vi "DHT11 Example.vi"() -> ()   [LabVIEW 2009, in "DHTXX.lvlib"]
uses:
  DHTXX.lvlib
  <vilib>/LabVIEW Interface for Arduino/LabVIEW Interface for Arduino.lvlib
panel:
  out "OK":bool
  in  "stop":bool
  out "Relative Humidity (%)":dbl(slide)
  out "Temperature (°C)":dbl(slide)
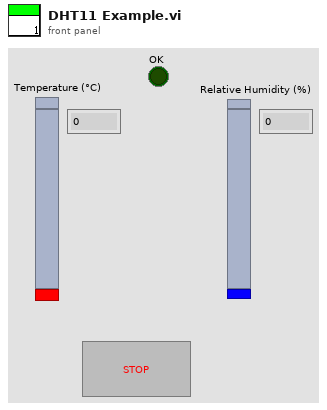
[diagram p1: front panel]
types:
  T1 = typedef "LabVIEW Interface for Arduino.lvlib/Arduino Resource.ctl" = cluster{"VISA resource":refnum<visa-resource-name>, "Board Type":T2, "Connection Type":enum8{"USB / Serial"}, "Bytes Per Packet (15)":u8}
  T2 = typedef "LabVIEW Interface for Arduino.lvlib/Board Type.ctl" = enum16{"Uno", "Dimuelanove w/Atmega 328", "Mega 2560"}
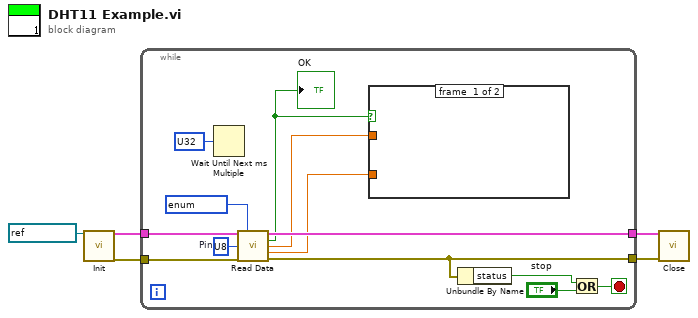
[diagram p0: block diagram]
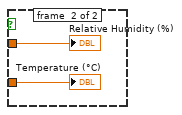
[diagram p2: hidden frame]
diagram:
  n1 = call <vilib>:"Init.vi"("VISA resource"=refnum<visa-resource-name> ?) -> ("Arduino Resource"=w5:T1, "error out"=w4:errorcluster)  [unwired: 17 in]
  n2 = while {
    tunnel: w5 -> [w18]
    tunnel: w4 -> [w17]
    tunnel: [w16] -> w3
    tunnel: [w8] -> w2
    stop <- w12 stop-if-true
    w9 = u8 ?  # Pin
    n3 = Wait Until Next ms Multiple(millisecond multiple=u32 ?) -> ()  [unwired: 1 out]
    n4 = call "Read Data.vi"("Arduino Resource"=w18, "Sensor Type"=enum16{"DHT11", "DHT21", "DHT22"} ?, "Pin"=w9, "error in (no error)"=w17) -> ("Arduino Resource"=w16:T1, "Successful?"=w15:bool, "Relative Humidity"=w14:dbl, "Temperature (°C)"=w13:dbl, "error out"=w8:errorcluster)  [unwired: 7 in]
    "OK" <- w15
    n5 = case shown="True" w15 {
      tunnel: w14 -> [_ w19]
      tunnel: w13 -> [_ w20]
      frame #0 {
      }
      frame #1 {
        "Relative Humidity (%)" <- w19
        "Temperature (°C)" <- w20
      }
    }
    n6 = Unbundle By Name(w8) -> ("status"=w7:bool)
    n7 = Or(x=w7, y="stop") -> (x .or. y?=w12:bool)
  }
  n8 = call <vilib>:"Close.vi"("Arduino Resource"=w3, "error in"=w2) -> ()  [unwired: 13 in, 1 out]
